vi "Query Trend Plot Parameters.vi"(0 "VISA resource name":refnum<visa-resource-name>, 5 "Channel Number (1: Trend Plot 1)":i32(ring)=1 items=["Trend Plot 1"=1, "Trend Plot 2"=2], 11 "error in (no error)":errorcluster) -> (1 "Units":string, 2 "Average Value":dbl, 3 "Minimum Value":dbl, 4 "VISA resource name out":refnum<visa-resource-name>, 6 "Maximum Value":dbl, 8 "Minimum Scale":dbl, 10 "Maximum Scale":dbl, 13 "Elapsed Time":string, 14 "Scale":dbl, 15 "error out":errorcluster)   [LabVIEW 2017, in "Tektronix TDS 200 1000 2000 Series.lvlib"]
doc: "Returns trend plot parameters corresponding to the selected channel.\n\n<b>Note(s):</b>\nThis VI is only applicable for TBS1000B series models."
uses:
  Tektronix TDS 200 1000 2000 Series.lvlib
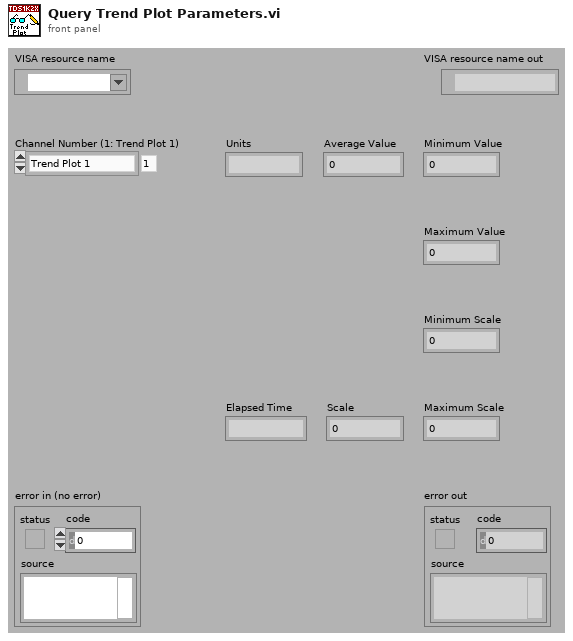
[diagram p1: front panel]
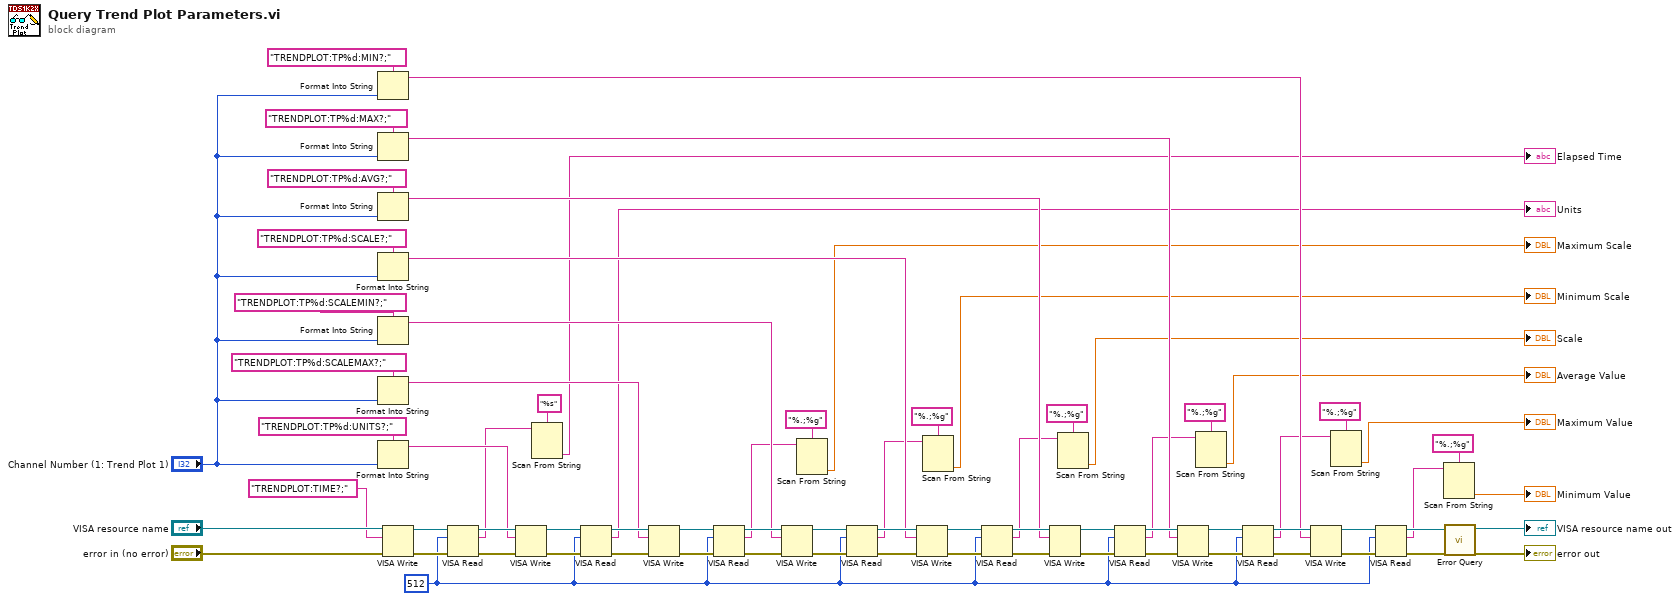
[diagram p0: block diagram]
diagram:
  w35 = u32 512 ("byte count")
  n1 = Format Into String(format string="TRENDPLOT:TP%d:MIN?;", "Channel Number (1: Trend Plot 1)") -> (resulting string=w23:string)  [unwired: 2 in, 1 out]
  n2 = Format Into String(format string="TRENDPLOT:TP%d:MAX?;", "Channel Number (1: Trend Plot 1)") -> (resulting string=w24:string)  [unwired: 2 in, 1 out]
  n3 = Format Into String(format string="TRENDPLOT:TP%d:AVG?;", "Channel Number (1: Trend Plot 1)") -> (resulting string=w25:string)  [unwired: 2 in, 1 out]
  n4 = Format Into String(format string="TRENDPLOT:TP%d:SCALE?;", "Channel Number (1: Trend Plot 1)") -> (resulting string=w26:string)  [unwired: 2 in, 1 out]
  n5 = Format Into String(format string="TRENDPLOT:TP%d:SCALEMIN?;", "Channel Number (1: Trend Plot 1)") -> (resulting string=w27:string)  [unwired: 2 in, 1 out]
  n6 = Format Into String(format string="TRENDPLOT:TP%d:SCALEMAX?;", "Channel Number (1: Trend Plot 1)") -> (resulting string=w28:string)  [unwired: 2 in, 1 out]
  n7 = Format Into String(format string="TRENDPLOT:TP%d:UNITS?;", "Channel Number (1: Trend Plot 1)") -> (resulting string=w30:string)  [unwired: 2 in, 1 out]
  n8 = VISA Write(VISA resource name="VISA resource name", write buffer="TRENDPLOT:TIME?;", error in (no error)="error in (no error)") -> (VISA resource name out=w63:refnum<visa-resource-name>, error out=w62:errorcluster)  [unwired: 1 out]
  n9 = VISA Read(VISA resource name=w63, byte count=w35, error in (no error)=w62) -> (VISA resource name out=w60:refnum<visa-resource-name>, read buffer=w2:string, error out=w59:errorcluster)  [unwired: 1 out]
  n10 = VISA Write(VISA resource name=w60, write buffer=w30, error in (no error)=w59) -> (VISA resource name out=w58:refnum<visa-resource-name>, error out=w61:errorcluster)  [unwired: 1 out]
  n11 = Scan From String(format string="%s", input string=w2) -> (output 1=→"Elapsed Time":string)  [unwired: 2 in, 4 out]
  n12 = VISA Read(VISA resource name=w58, byte count=w35, error in (no error)=w61) -> (VISA resource name out=w51:refnum<visa-resource-name>, read buffer=→"Units":string, error out=w50:errorcluster)  [unwired: 1 out]
  n13 = VISA Write(VISA resource name=w51, write buffer=w28, error in (no error)=w50) -> (VISA resource name out=w57:refnum<visa-resource-name>, error out=w56:errorcluster)  [unwired: 1 out]
  n14 = VISA Read(VISA resource name=w57, byte count=w35, error in (no error)=w56) -> (VISA resource name out=w54:refnum<visa-resource-name>, read buffer=w6:string, error out=w53:errorcluster)  [unwired: 1 out]
  n15 = VISA Write(VISA resource name=w54, write buffer=w27, error in (no error)=w53) -> (VISA resource name out=w52:refnum<visa-resource-name>, error out=w55:errorcluster)  [unwired: 1 out]
  n16 = Scan From String(format string="%.;%g", input string=w6) -> (output 1=→"Maximum Scale":dbl)  [unwired: 2 in, 4 out]
  n17 = VISA Read(VISA resource name=w52, byte count=w35, error in (no error)=w55) -> (VISA resource name out=w43:refnum<visa-resource-name>, read buffer=w9:string, error out=w42:errorcluster)  [unwired: 1 out]
  n18 = VISA Write(VISA resource name=w43, write buffer=w26, error in (no error)=w42) -> (VISA resource name out=w49:refnum<visa-resource-name>, error out=w48:errorcluster)  [unwired: 1 out]
  n19 = Scan From String(format string="%.;%g", input string=w9) -> (output 1=→"Minimum Scale":dbl)  [unwired: 2 in, 4 out]
  n20 = VISA Read(VISA resource name=w49, byte count=w35, error in (no error)=w48) -> (VISA resource name out=w46:refnum<visa-resource-name>, read buffer=w12:string, error out=w45:errorcluster)  [unwired: 1 out]
  n21 = VISA Write(VISA resource name=w46, write buffer=w25, error in (no error)=w45) -> (VISA resource name out=w44:refnum<visa-resource-name>, error out=w47:errorcluster)  [unwired: 1 out]
  n22 = Scan From String(format string="%.;%g", input string=w12) -> (output 1=→"Scale":dbl)  [unwired: 2 in, 4 out]
  n23 = VISA Read(VISA resource name=w44, byte count=w35, error in (no error)=w47) -> (VISA resource name out=w34:refnum<visa-resource-name>, read buffer=w15:string, error out=w33:errorcluster)  [unwired: 1 out]
  n24 = VISA Write(VISA resource name=w34, write buffer=w24, error in (no error)=w33) -> (VISA resource name out=w41:refnum<visa-resource-name>, error out=w40:errorcluster)  [unwired: 1 out]
  n25 = Scan From String(format string="%.;%g", input string=w15) -> (output 1=→"Average Value":dbl)  [unwired: 2 in, 4 out]
  n26 = VISA Read(VISA resource name=w41, byte count=w35, error in (no error)=w40) -> (VISA resource name out=w38:refnum<visa-resource-name>, read buffer=w18:string, error out=w37:errorcluster)  [unwired: 1 out]
  n27 = VISA Write(VISA resource name=w38, write buffer=w23, error in (no error)=w37) -> (VISA resource name out=w36:refnum<visa-resource-name>, error out=w39:errorcluster)  [unwired: 1 out]
  n28 = Scan From String(format string="%.;%g", input string=w18) -> (output 1=→"Maximum Value":dbl)  [unwired: 2 in, 4 out]
  n29 = VISA Read(VISA resource name=w36, byte count=w35, error in (no error)=w39) -> (VISA resource name out=w32:refnum<visa-resource-name>, read buffer=w22:string, error out=w31:errorcluster)  [unwired: 1 out]
  n30 = Scan From String(format string="%.;%g", input string=w22) -> (output 1=→"Minimum Value":dbl)  [unwired: 2 in, 4 out]
  n31 = call "Error Query.vi"("error in (no error)"=w31, "VISA resource name"=w32) -> ("error out"=→"error out":errorcluster, "VISA resource name out"=→"VISA resource name out":refnum<visa-resource-name>)  [unwired: 8 out]
